vi "DSF.Engine.Memory.ObjectPool.Get Object.vi"(8 "error in (no error)":errorcluster, 10 "index":i32, 11 "ObjectPool in":refnum<class "DSF.Engine.Memory.ObjectPool.lvclass">) -> (0 "error out":errorcluster, 1 "Object":refnum<class>, 3 "ObjectPool out":refnum<class "DSF.Engine.Memory.ObjectPool.lvclass">)   [LabVIEW 2016, in "DSF.Engine.lvlib" / "DSF.Engine.Memory.ObjectPool.lvclass"]
uses:
  DSF.Engine.Memory.ObjectPool.lvclass
  DSF.Engine.Memory.ObjectPool.lvclass/DSF.Engine.Memory.ObjectPool.ctl
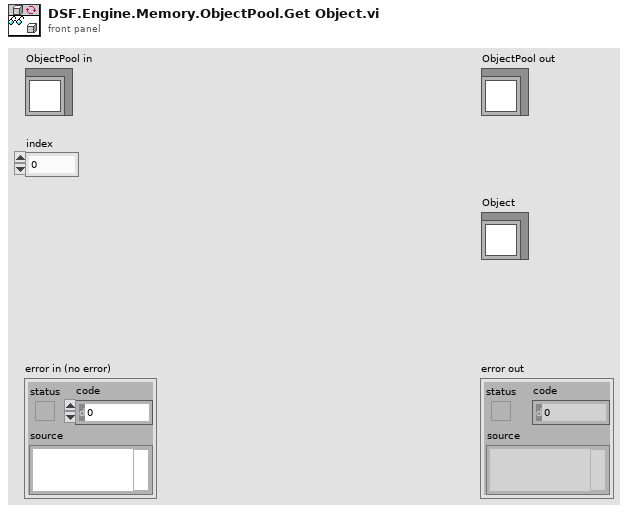
[diagram p1: front panel]
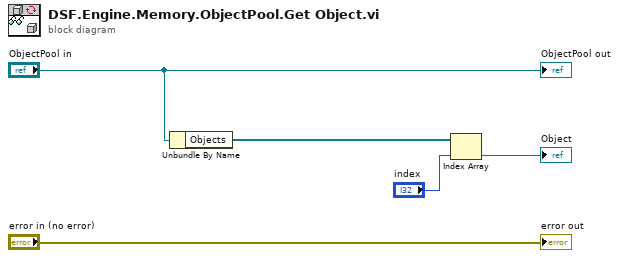
[diagram p0: block diagram]
diagram:
  n1 = Unbundle By Name("ObjectPool in") -> ("Objects"=w2:refnum<class>[])
  n2 = Index Array(array=w2, index="index") -> (element=→"Object":refnum<class>)
  "error out" <- "error in (no error)"
  "ObjectPool out" <- "ObjectPool in"
